vi "Get Supported Subdevices.vi"(8 "error in (no error)":errorcluster) -> (0 "error out":errorcluster, 3 "devices supported":i32)   [LabVIEW 2013]
uses:
  libkinect_wrapper.dll
panel:
  # "7 = all\n3 = motor and camera\n1 = motor"
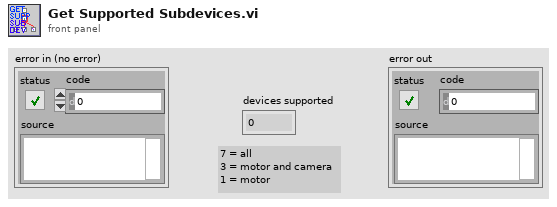
[diagram p1: front panel]
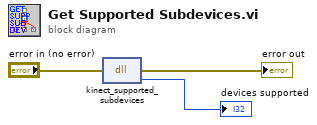
[diagram p0: block diagram]
diagram:
  n1 = dll-call lib="libkinect_wrapper.*" fn="kinect_supported_subdevices"(error in="error in (no error)") -> (error out=→"error out":errorcluster, "return type"=→"devices supported":i32)  [unwired: 2 in, 1 out]
